vi "SetPxx.vi"(6 "Legacy (f)?":bool, 8 "error in (no error)":errorcluster, 10 "SetPxx":T1) -> (0 "error out":errorcluster)   [LabVIEW 2011]
uses:
  PIM Parameters.ctl
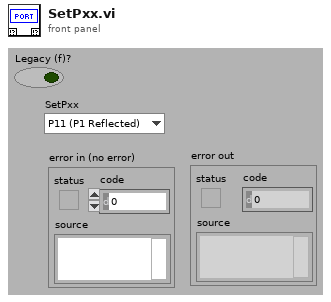
[diagram p1: front panel]
types:
  T1 = typedef "PIM Parameters.ctl" = enum16{"P11 (P1 Reflected)", "P12 (P2 Through)", "P21 (P1 Through)", "P22 (P2 Reflected)"}
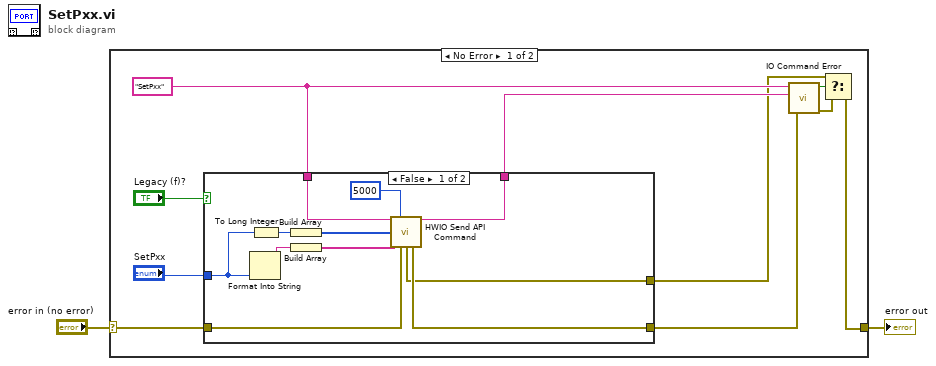
[diagram p0: block diagram]
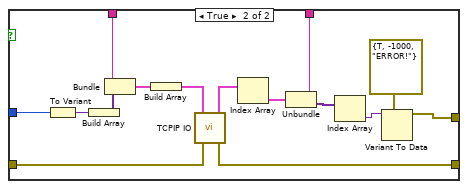
[diagram p2: hidden frame]
diagram:
  n1 = case shown="No Error" "error in (no error)" {
    selector: "error in (no error)" -> [w8 w39]
    tunnel: [w4 w39] -> w2
    frame No Error {
      w10 = "SetPxx"
      n2 = case shown="False" "Legacy (f)?" {
        tunnel: "SetPxx" -> [w17 w36]
        tunnel: [w21 w33] -> w11
        tunnel: w10 -> [w20 w32]
        tunnel: [w22 w31] -> w9
        tunnel: w8 -> [w23 w28]
        tunnel: [w14 w25] -> w7
        frame False {
          n3 = Format Into String(w17) -> (resulting string=w16:string)  [unwired: 3 in, 1 out]
          n4 = To Long Integer(number=w17) -> (32bit integer=w18:i32)
          n5 = Build Array(w18) -> (w19:i32[])
          n6 = Build Array(w16) -> (w15:string[])
          n7 = call "HWIO Send API Command.vi"("Action"=w20, "Timeout ms (5000)"=5000 ("PerCommand Timeout (ms)"), "Integer"=w19, "String"=w15, "error in (no error)"=w23) -> ("Action out"=w21:string, "HWError"=w14:errorcluster, "error out"=w22:errorcluster)  [unwired: 3 in, 5 out]
        }
        frame True {
          n8 = To Variant(anything=w36) -> (Variant=w38:variant)
          n9 = Build Array(w38) -> (w37:variant[])
          n10 = Bundle(w32, w37) -> (w34:cluster{string, variant[]})  [unwired: 1 out]
          n11 = Build Array(w34) -> (w35:cluster{string, variant[]}[])
          n12 = call "TCPIP IO.vi"("error in (no error)"=w28, "Commands"=w35) -> ("error out"=w31:errorcluster, "Responses"=w29:cluster{string, variant[]}[])  [unwired: 1 in, 3 out]
          n13 = Index Array(array=w29) -> (element=w30:cluster{string, variant[]})  [unwired: 1 in]
          n14 = Unbundle(w30) -> (w33:string, w24:variant[])
          n15 = Index Array(array=w24) -> (element=w27:variant)  [unwired: 1 in]
          n16 = Variant To Data(type=errorcluster {"status"=TRUE, "code"=-1000, "source"="ERROR!"} ("error out"), Variant=w27) -> (data=w25:errorcluster)  [unwired: 1 in, 1 out]
        }
      }
      n17 = call "IO Command Error.vi"("error in (no error)"=w9, "Command Returned (\"\")"=w11, "Command Sent (\"\")"=w10) -> ("error out"=w5:errorcluster, "HW ERR?"=w6:bool)  [unwired: 3 out]
      n18 = Select(t=w7, s=w6, f=w5) -> (s? t:f=w4:errorcluster)
    }
    frame Error {
    }
  }
  "error out" <- w2
